vi "UDP_set_receive_buffer.vi"(7 "error in (no error)":errorcluster, 8 "Receive Buffer Size":u32=8192, 10 "connection ID":refnum<k16>) -> (0 "error out":errorcluster, 3 "connection ID out":refnum<k16>)   [LabVIEW 2018]
doc: "This VI sets the receive buffer size for a given UDP socket connection."
uses:
  wsock32.dll
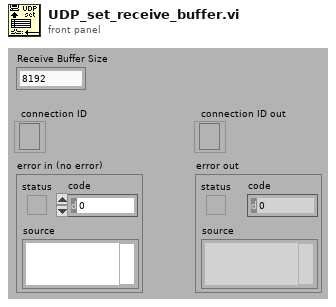
[diagram p1: front panel]
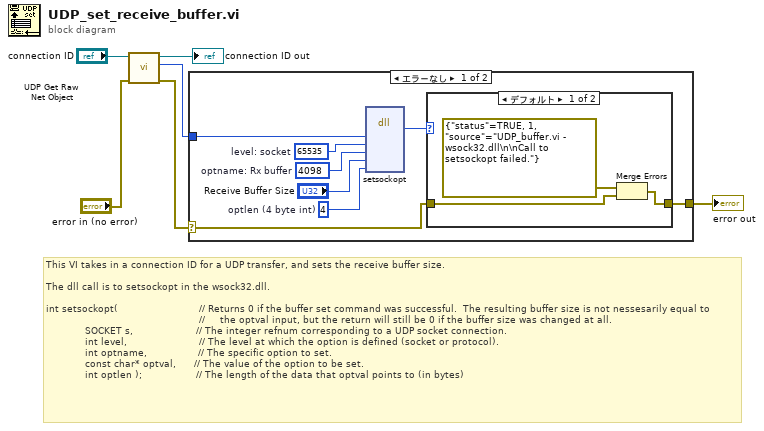
[diagram p0: block diagram]
diagram:
  # "This VI takes in a connection ID for a UDP transfer, and sets the receive buffer size.\n\nThe dll call is to setsockopt in the wsock32.dll.\n\nint setsockopt(                           // Returns 0 if the buffer set command was successful.  The resulting buffer size is not nessesarily equal to\n                                                   //     the optval input, but the return will still be 0 if the buffer size was changed at all. \n             SOCKET s,                     // The integer refnum corresponding to a UDP socket connection.     \n             int level,                        // The level at which the option is defined (socket or protocol). \n             int optname,                 // The specific option to set.\n             const char* optval,      // The value of the option to be set.\n             int optlen );                  // The length of the data that optval points to (in bytes)"
  n1 = call <vilib>:"UDP Get Raw Net Object.vi"("error in (no error)"="error in (no error)", "connection ID"="connection ID") -> ("error out"=w6:errorcluster, "raw net object"=w3:u64, "connection ID out"=→"connection ID out":refnum<k16>)  [unwired: 7 in]
  n2 = case shown="エラーなし" w6 {
    selector: w6 -> [w7 w19]
    tunnel: [w10 w19] -> w2
    tunnel: w3 -> [w9 _]
    frame No Error {
      w12 = 4  # optlen (4 byte int)
      w13 = 4098  # optname: Rx buffer
      w14 = 65535  # level: socket
      n3 = dll-call lib="wsock32.dll" fn="setsockopt" ("Call Library Function")("socket"=w9, "protocol"=w14, "selector"=w13, "value"="Receive Buffer Size", "size"=w12) -> ("return type"=w11:i32)  [unwired: 8 in, 2 out]
      n4 = case shown="デフォルト" w11 {
        tunnel: [w17 w18] -> w10
        tunnel: w7 -> [w15 w18]
        frame Default {
          n5 = Merge Errors(cluster{"status":bool, i32, "source":string} {"status"=TRUE, 1, "source"="UDP_buffer.vi - wsock32.dll\n\nCall to setsockopt failed."} ("error out"), w15) -> (w17:errorcluster)
        }
        frame 0 {
        }
      }
    }
    frame Error {
    }
  }
  "error out" <- w2
